vi "Replace comas for cr.vi"(8 "Tokens to replace":map{string, string}(c390), 10 "Col to Replace CR":i32=1, 11 "Array in":string[][](array[string])) -> (3 "Array Replaced":string[][](array[string]))   [LabVIEW 2019, in "Panther Dashboard.lvlib"]
uses:
  Panther Dashboard.lvlib
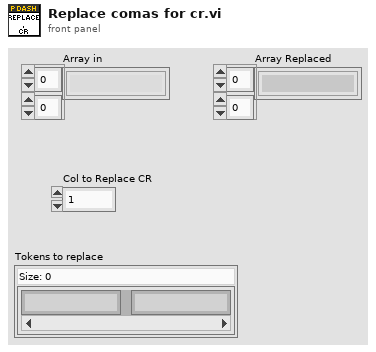
[diagram p1: front panel]
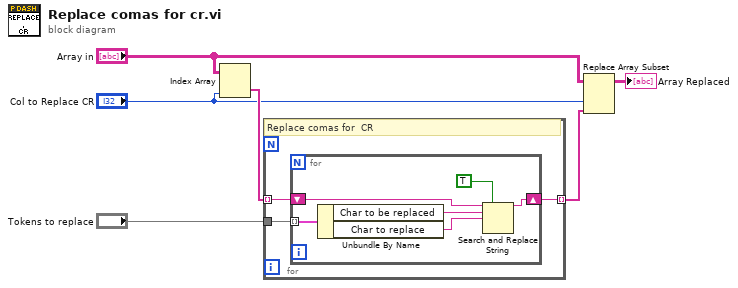
[diagram p0: block diagram]
diagram:
  n1 = Index Array(array="Array in", index (col)="Col to Replace CR") -> (element=w6:string[])  [unwired: 1 in]
  n2 = for {
    tunnel: w6 -> [w9] mode=indexing
    tunnel: [w8] -> w4 mode=indexing
    tunnel: "Tokens to replace" -> [w7]
    # "Replace comas for  CR"
    n3 = for {
      shift-right: [w13] -> w8
      shift-left: w9 -> [w15]
      tunnel: w7 -> [w12] mode=indexing
      n4 = Unbundle By Name(w12) -> ("Char to be replaced"=w11:string, "Char to replace"=w10:string)
      n5 = Search and Replace String(replace all?=TRUE ("replace all? (F)"), input string=w15, search string=w11, replace string=w10) -> (result string=w13:string)  [unwired: 4 in, 3 out]
    }
  }
  n6 = Replace Array Subset(array="Array in", new element=w4, index (col)="Col to Replace CR") -> (→"Array Replaced":string[][])  [unwired: 1 in]
